vi "Write UTC Time For String Format.vi"(8 "error in (no error)":errorcluster, 10 "UTC Time For String Format":bool, 11 "Time in":refnum<class "Abs_Time.lvclass">) -> (0 "error out":errorcluster, 3 "Time out":refnum<class "Abs_Time.lvclass">)   [LabVIEW 2021, in "Abs_Time.lvclass"]
uses:
  Abs_Time.lvclass
  Abs_Time.lvclass/Abs_Time.ctl
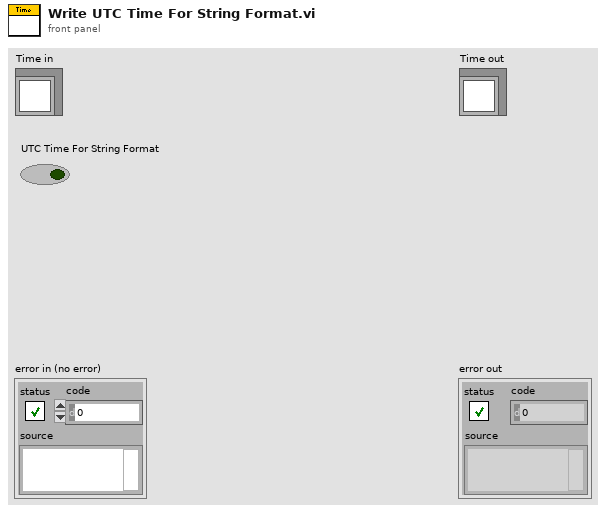
[diagram p1: front panel]
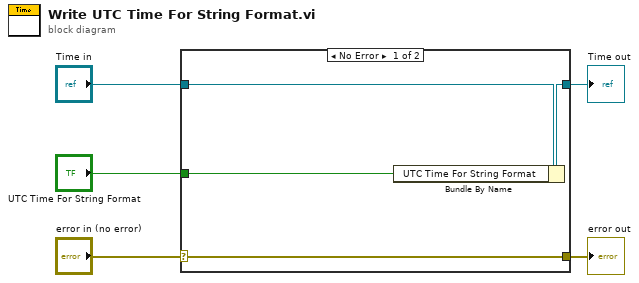
[diagram p0: block diagram]
diagram:
  n1 = case shown="No Error" "error in (no error)" {
    selector: "error in (no error)" -> [w9 w10]
    tunnel: [w9 w10] -> w4
    tunnel: [w7 w11] -> w2
    tunnel: "Time in" -> [w8 w11]
    tunnel: "UTC Time For String Format" -> [w6 _]
    frame No Error {
      n2 = Bundle By Name(cluster=w8, "UTC Time For String Format"=w6) -> (w7:refnum<class "Abs_Time.lvclass">)
    }
    frame Error {
    }
  }
  "error out" <- w4
  "Time out" <- w2
